vi "Config FX Set.vi"(5 "Max # Of Tries":i32, 6 "Send Cmd Timout(ms)":u32=300, 8 "Error":errorcluster, 9 "Wrist Config":T6={"WristHW Ver"=0, "CAN"={"ID"=0, "Bus"=""}, "Output"={"Type"=enum."Counter-Clockwise", "Neutral"=enum."EEPROMSetting", "Max"={"FWD"=0.0, "REV"=-1.0}, "Min"={"FWD"=0.0, "REV"=0.0}, "OL Ramp Rate (S)"=0.0, "Dead Band"=0.0}, "CL"={"Gains"={"P"=1.0, "I"=0.01, "D"=0.0, "F"=0.0}, "Error Allowed"={"High"=0.0, "Low"=0.0}, "I Zone"={"High"=10000.0, "Low"=-1000.0}, "Max Out"={"FWD"=1.0, "REV"=-1.0}, "Max I Accu"={"High"=10.0, "Low"=-10.0}, "CL Ramp Rate (S)"=0.0}, "MM"={"Cruise Velocity"=5000, "Acceleration"=5000}, "TravelLimits"={"Hard"={"FWD Switch Normal"=enum."Normally Open", "FWD On will Zero Encoder "=FALSE, "REV Switch Normal"=enum."Normally Open", "REV On will Zero Encoder "=FALSE}, "Soft"={"FWD"={"Enable"=FALSE, "Counts"=0}, "REV"={"Enable"=FALSE, "Counts"=0}}}, "Cancoder"={"ID"=0, "CW(t) CCW(f)"=TRUE, "Zero Offset"=0.0}, "CurrentLimit"={"Enable"=FALSE, "Current Limit"=0.0, "Threshold Current"=0.0, "Threshold Time"=0.0}} {"TravelLimits"."Soft"."REV"."Counts" format="%#.0f"; "TravelLimits"."Soft"."FWD"."Counts" format="%#.0f"; "Output"."Min"."REV" format="%.2f"; "Output"."Min"."FWD" format="%.2f"; "Output"."Max"."REV" format="%.2f"; "Output"."Max"."FWD" format="%.2f"; "CL"."Max I Accu"."Low" format="%#.8f"; "CL"."Max I Accu"."High" format="%#.8f"; "CL"."Gains"."F" format="%#.8f"; "CL"."Gains"."D" format="%#.8f"; "CL"."Gains"."I" format="%#.8f"; "CL"."Gains"."P" format="%#.8f"; "CL"."Error Allowed"."Low" format="%#.8f"; "CL"."Error Allowed"."High" format="%#.8f"; "CL"."I Zone"."Low" format="%#.8f"; "CL"."I Zone"."High" format="%#.8f"; "CL"."Max Out"."REV" format="%.2f"; "CL"."Max Out"."FWD" format="%.2f"}, 11 "PhoenixMotorControlDevRef":T1={"DeviceStatus"={"status"=FALSE, "code"=0, "source"=""}, "Type"=enum."PWM", "PWM"={"PWM Channel"=enum."Invalid", "DeadBand"={"Name"="", "maxPositivePwm"=0, "minPositivePwm"=0, "centerPwm"=0, "maxNegativePwm"=0, "minNegativePwm"=0, "angularRange"=0}}, "CAN"={"Device Number"=0, "SetOutput VI Ref"=variant, "GetOutput VI Ref"=variant, "Enable VI Ref"=variant, "Disable VI Ref"=variant, "Data"=variant}, "Invert"=FALSE, "DIO PWM"={"PWM \"Enable\" Channel"=enum."Invalid", "DIOChannel"=enum."Invalid", "PWM Rate"=0.0}}) -> (0 "Error Out":errorcluster, 3 "PhoenixMotorControlDevRef Out Out":T1)   [LabVIEW 2023, in "Wrist_ACT.lvlib"]
uses:
  Wrist_ACT.lvlib
  <vilib>/Utility/Data Type/NI_Data Type.lvlib
  Shared Code/TypeDefs/Cluser_CAN Data.ctl
  <vilib>/Rock Robotics/WPI/ThirdParty/Phoenix-LabVIEW/Motor Controller/Controls/CTRE_Phoenix_MotorControl_TalonFXInvertType.ctl
  <vilib>/Rock Robotics/WPI/ThirdParty/Phoenix-LabVIEW/Motor Controller/Controls/CTRE_Phoenix_MotorControl_NeutralMode.ctl
  Shared Code/TypeDefs/Cluster_FWD  REV Values.ctl
  Shared Code/TypeDefs/Cluster_Config Motor Output.ctl
  Shared Code/TypeDefs/Cluster_PID Gains.ctl
  Shared Code/TypeDefs/Cluster_High-Low.ctl
  Shared Code/TypeDefs/Cluster_PID Config.ctl
  Shared Code/TypeDefs/Cluster_Motion Magic Parameters.ctl
  <vilib>/Rock Robotics/WPI/ThirdParty/Phoenix-LabVIEW/Motor Controller/Controls/CTRE_Phoenix_MotorControl_LimitSwitchNormal.ctl
  Shared Code/TypeDefs/Cluser_Hard Limits.ctl
  Shared Code/TypeDefs/Cluser_Enable-Value I32.ctl
  Shared Code/TypeDefs/Cluser_Config_Soft Limits.ctl
  Shared Code/TypeDefs/Cluser_Limit Travel Config.ctl
  <vilib>/Rock Robotics/WPI/ThirdParty/Phoenix-LabVIEW/Motor Controller/Controls/CTRE_Phoenix_MotorControl_RemoteSourceType.ctl
  <vilib>/Rock Robotics/WPI/ThirdParty/Phoenix-LabVIEW/Motor Controller/Controls/CTRE_Phoenix_MotorControl_FeedbackDevice_TalonFX.ctl
  Shared Code/TypeDefs/Cluster_Config FX Motor Output.ctl
  Shared Code/TypeDefs/Cluster_FX SLOT PID Config.ctl
  <vilib>/Rock Robotics/SystemInterfaces/DIO/FPGA_DIOPWMChannel.ctl
  <vilib>/Rock Robotics/WPI/PWM/WPI_PWMDeadband.ctl
  <vilib>/Rock Robotics/WPI/MotorControl/WPI_MotorControlType.ctl
  <vilib>/Rock Robotics/SystemInterfaces/DIO/FPGA_DIOChannel.ctl
  <vilib>/Rock Robotics/WPI/MotorControl/WPI_MotorControlDeviceRef.ctl
  Shared Code/TypeDefs/Cluster_Wrist_Config HW Values.ctl
  Shared Code/TypeDefs/Cluster_Config_Cancoder Data.ctl
  Shared Code/TypeDefs/Cluser_Config_Current Limits.ctl
panel:
  # "Tune Output\nto 1023 Max"
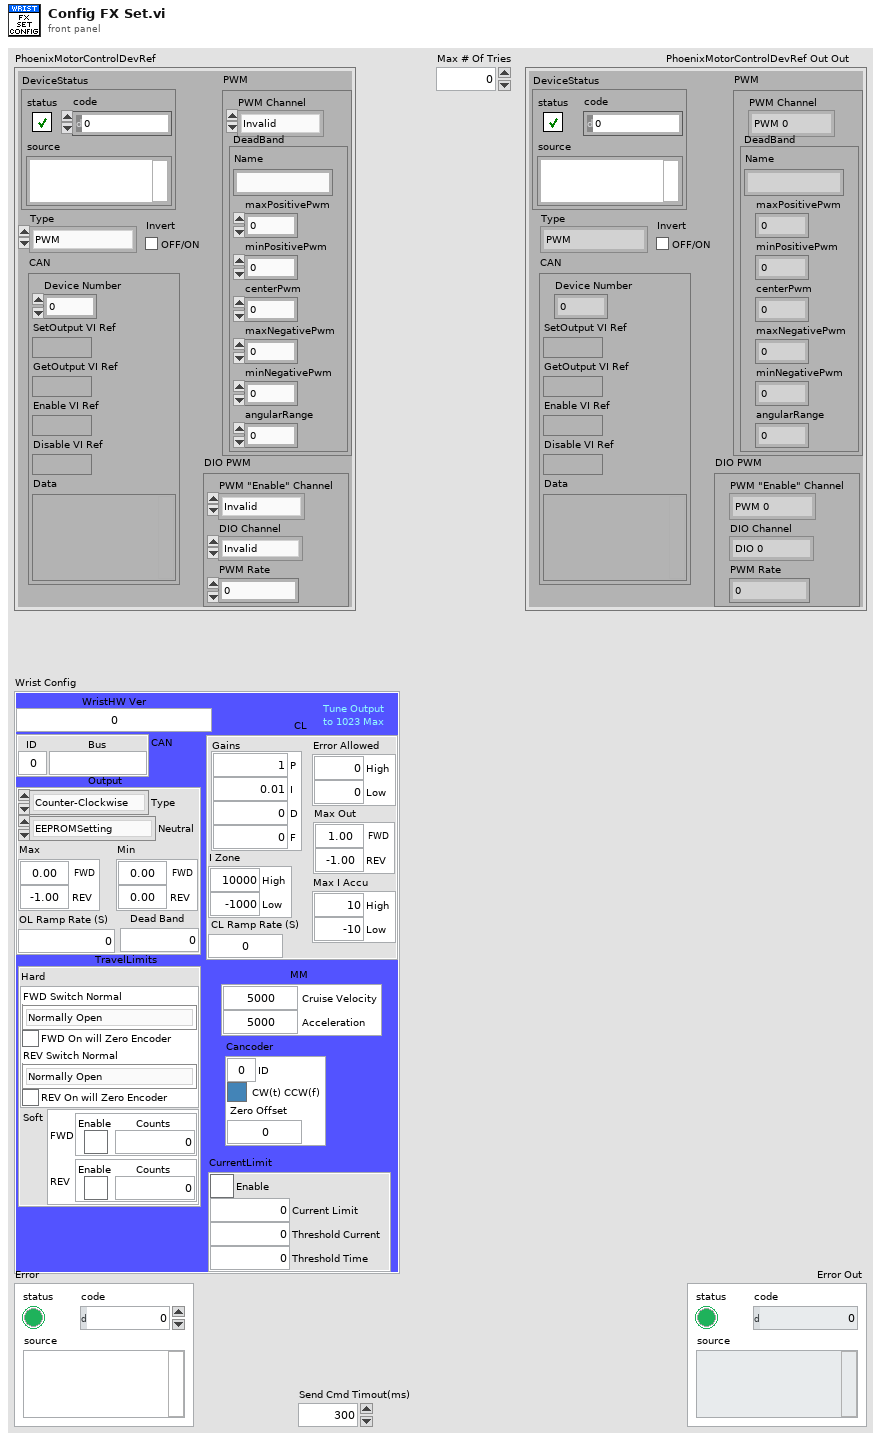
[diagram p1: front panel]
types:
  T1 = typedef "WPI_MotorControlDeviceRef.ctl" = cluster{"DeviceStatus":errorcluster, "Type":T2, "PWM":cluster{"PWM Channel":T3, "DeadBand":T4}, "CAN":cluster{"Device Number":u8, "SetOutput VI Ref":variant, "GetOutput VI Ref":variant, "Enable VI Ref":variant, "Disable VI Ref":variant, "Data":variant}, "Invert":bool, "DIO PWM":cluster{"PWM \"Enable\" Channel":T3, "DIOChannel":T5, "PWM Rate":dbl}}
  T2 = typedef "WPI_MotorControlType.ctl" = enum16{"PWM", "CAN", "DIO PWM"}
  T3 = typedef "FPGA_DIOPWMChannel.ctl" = enum8{"PWM 0", "PWM 1", "PWM 2", "PWM 3", "PWM 4", "PWM 5", "PWM 6", "PWM 7", "PWM 8", "PWM 9", "PWM MXP 0", "PWM MXP 1", "PWM MXP 2", "PWM MXP 3", "PWM MXP 4", "PWM MXP 5", "PWM MXP 6", "PWM MXP 7", "PWM MXP 8", "PWM MXP 9", "Invalid"}
  T4 = typedef "WPI_PWMDeadband.ctl" = cluster{"Name":string, "maxPositivePwm":i32, "minPositivePwm":i32, "centerPwm":i32, "maxNegativePwm":i32, "minNegativePwm":i32, "angularRange":u16}
  T5 = typedef "FPGA_DIOChannel.ctl" = enum8{"DIO 0", "DIO 1", "DIO 2", "DIO 3", "DIO 4", "DIO 5", "DIO 6", "DIO 7", "DIO 8", "DIO 9", "DIO MXP 0", "DIO MXP 1", "DIO MXP 2", "DIO MXP 3", "DIO MXP 4", "DIO MXP 5", "DIO MXP 6", "DIO MXP 7", "DIO MXP 8", "DIO MXP 9", "DIO MXP 10", "DIO MXP 11", "DIO MXP 12", "DIO MXP 13", "DIO MXP 14", "DIO MXP 15", "SPI Port CS1", "SPI Port CS2", "SPI Port CS3", "SPI Port MISO", "SPI Port MOSI", "Invalid"}
  T6 = typedef "Cluster_Wrist_Config HW Values.ctl" = cluster{"WristHW Ver":u64, "CAN":T7, "Output":T8, "CL":T12, "MM":T15, "TravelLimits":T16, "Cancoder":T21, "CurrentLimit":T22}
  T7 = typedef "Cluser_CAN Data.ctl" = cluster{"ID":u8, "Bus":string}
  T8 = typedef "Cluster_Config Motor Output.ctl" = cluster{"Type":T9, "Neutral":T10, "Max":T11, "Min":T11, "OL Ramp Rate (S)":dbl, "Dead Band":dbl}
  T9 = typedef "CTRE_Phoenix_MotorControl_TalonFXInvertType.ctl" = enum16{"Counter-Clockwise", "Clockwise"}
  T10 = typedef "CTRE_Phoenix_MotorControl_NeutralMode.ctl" = enum8{"EEPROMSetting", "Override to Coast", "Override to Brake"}
  T11 = typedef "Cluster_FWD  REV Values.ctl" = cluster{"FWD":dbl, "REV":dbl}
  T12 = typedef "Cluster_PID Config.ctl" = cluster{"Gains":T13, "Error Allowed":T14, "I Zone":T14, "Max Out":T11, "Max I Accu":T14, "CL Ramp Rate (S)":dbl}
  T13 = typedef "Cluster_PID Gains.ctl" = cluster{"P":dbl, "I":dbl, "D":dbl, "F":dbl}
  T14 = typedef "Cluster_High-Low.ctl" = cluster{"High":dbl, "Low":dbl}
  T15 = typedef "Cluster_Motion Magic Parameters.ctl" = cluster{"Cruise Velocity":i32, "Acceleration":i32}
  T16 = typedef "Cluser_Limit Travel Config.ctl" = cluster{"Hard":T17, "Soft":T19}
  T17 = typedef "Cluser_Hard Limits.ctl" = cluster{"FWD Switch Normal":T18, "FWD On will Zero Encoder ":bool, "REV Switch Normal":T18, "REV On will Zero Encoder ":bool}
  T18 = typedef "CTRE_Phoenix_MotorControl_LimitSwitchNormal.ctl" = enum16{"Normally Open", "Normally Closed", "Disabled"}
  T19 = typedef "Cluser_Config_Soft Limits.ctl" = cluster{"FWD":T20, "REV":T20}
  T20 = typedef "Cluser_Enable-Value I32.ctl" = cluster{"Enable":bool, "Counts":i32}
  T21 = typedef "Cluster_Config_Cancoder Data.ctl" = cluster{"ID":u8, "CW(t) CCW(f)":bool, "Zero Offset":dbl}
  T22 = typedef "Cluser_Config_Current Limits.ctl" = cluster{"Enable":bool, "Current Limit":dbl, "Threshold Current":dbl, "Threshold Time":dbl}
  T23 = typedef "Cluster_FX SLOT PID Config.ctl" = cluster{"Gains":T13, "Error Allowed":dbl, "I Zone":dbl, "Peak Out 0-1":dbl, "Max I Accu":dbl}
  T24 = typedef "Cluster_Config FX Motor Output.ctl" = cluster{"Type":T9, "Neutral":T10, "Max":T11, "Min":T11, "OL Ramp Rate (S)":dbl, "Dead Band":dbl, "CL Ramp Rate (S)":dbl}
  T25 = typedef "CTRE_Phoenix_MotorControl_RemoteSourceType.ctl" = enum16{"Off", "Talon SRX Selected Sensor", "Pigeon IMU Yaw", "Pigeon IMU Pitch", "Pigeon IMU Roll", "CANifier Quadrature", "CANifier PWM Input 0", "CANifier PWM Input 1", "CANifier PWM Input 2", "CANifier PWM Input 3", "Gadgeteer Pigeon Yaw", "Gadgeteer Pigeon Pitch", "Gadgeteer Pigeon Roll", "CANCoder"}
  T26 = typedef "CTRE_Phoenix_MotorControl_FeedbackDevice_TalonFX.ctl" = i8
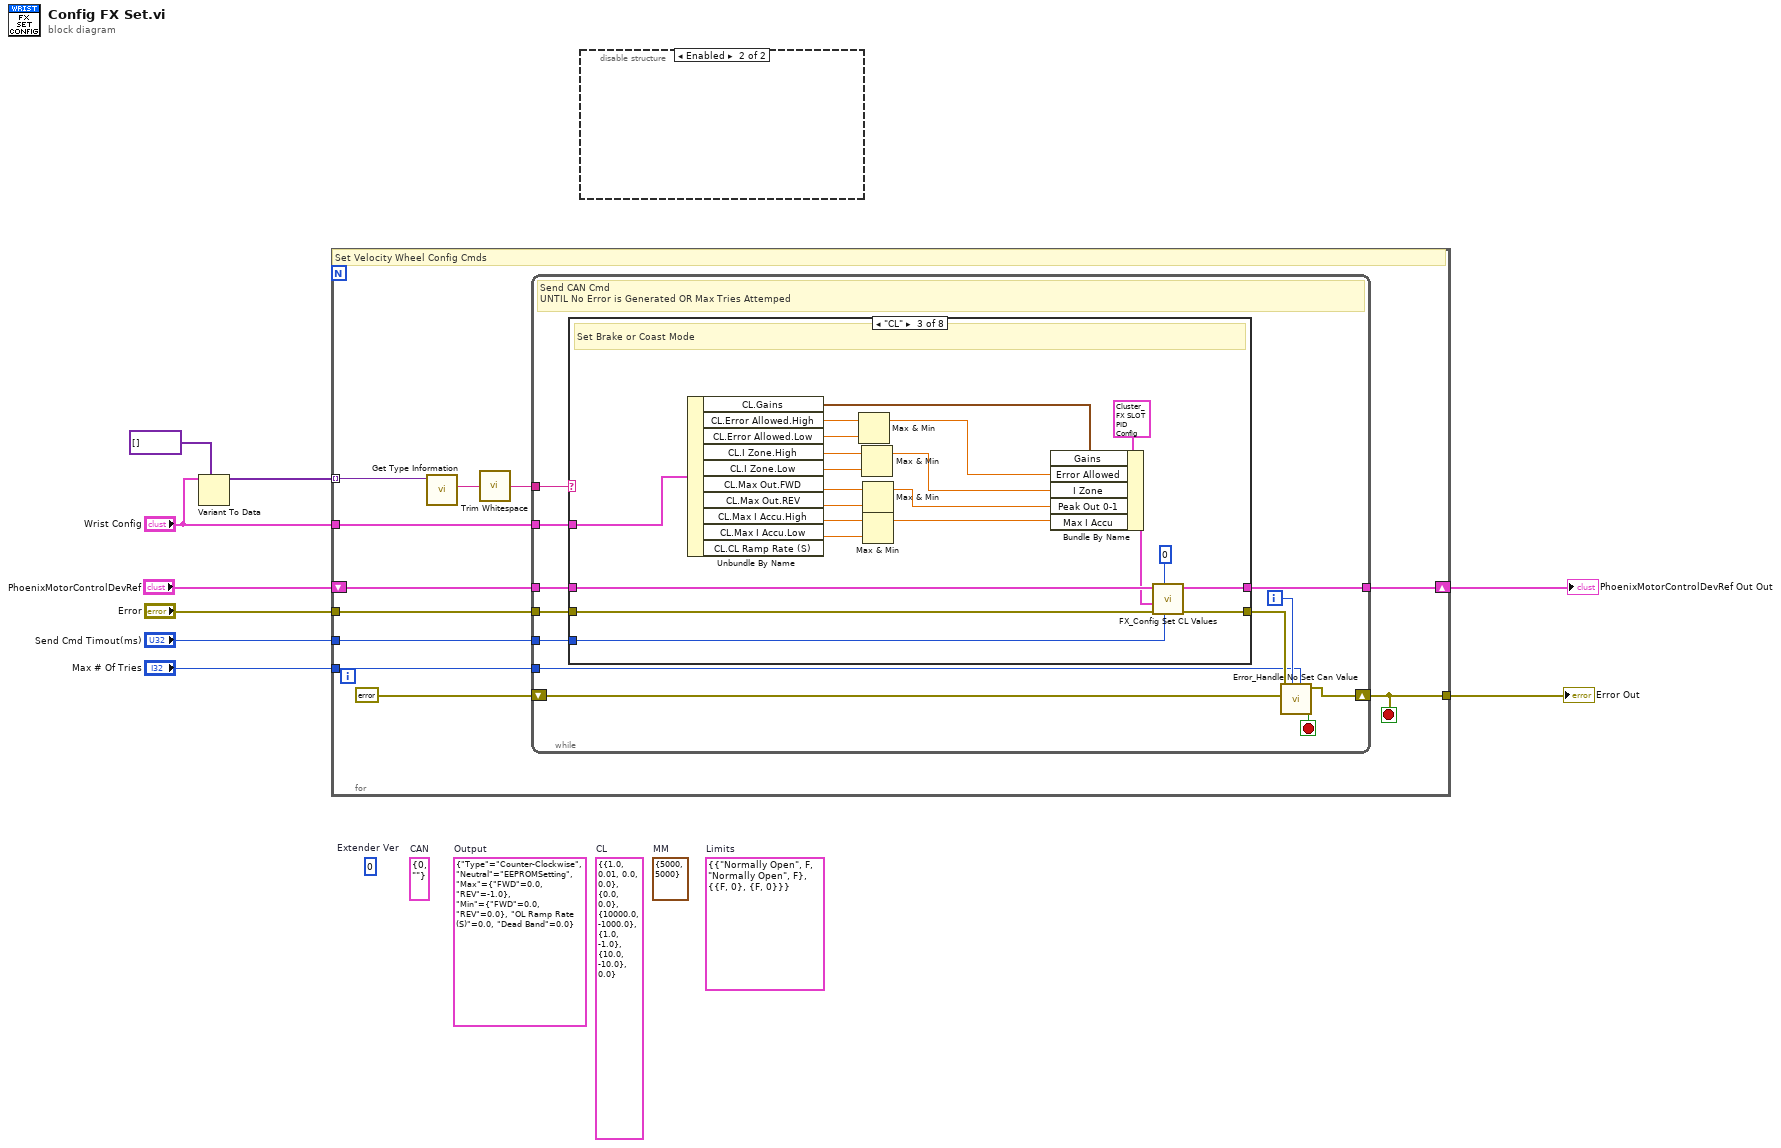
[diagram p0: block diagram]
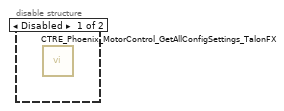
[diagram p2: hidden frame]
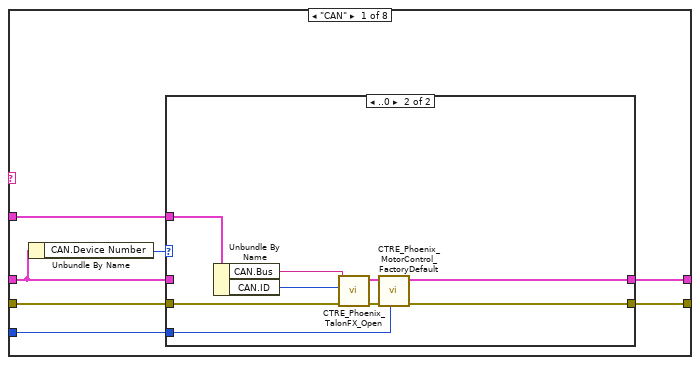
[diagram p3: hidden frame]
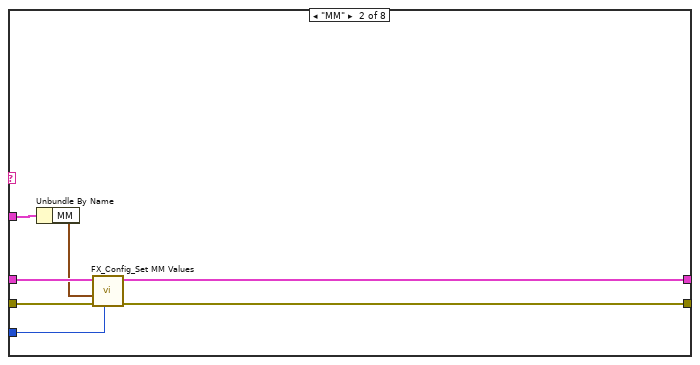
[diagram p5: hidden frame]
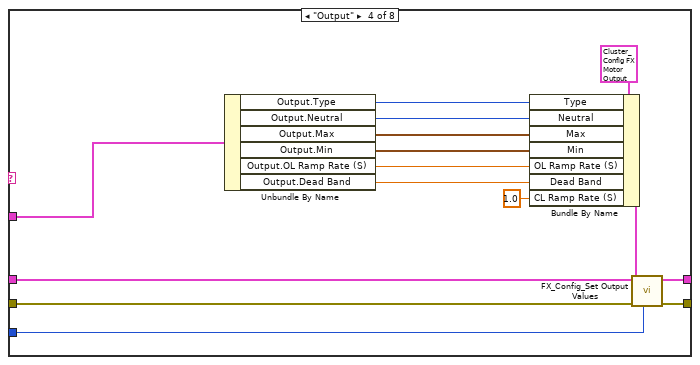
[diagram p6: hidden frame]
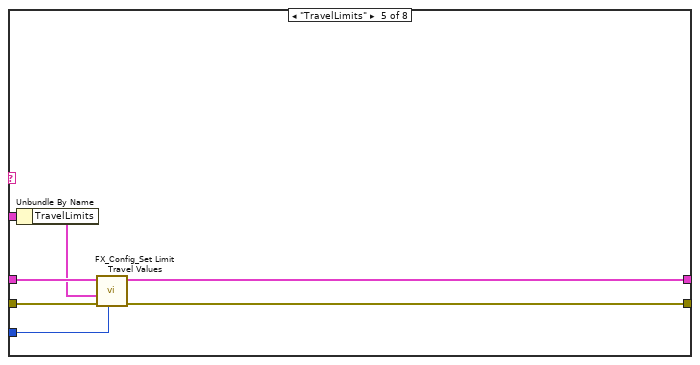
[diagram p7: hidden frame]
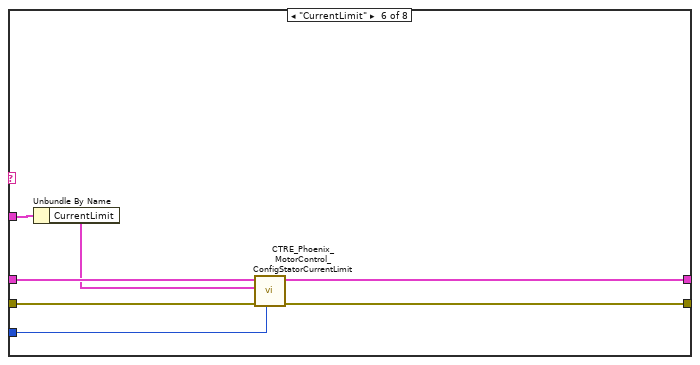
[diagram p8: hidden frame]
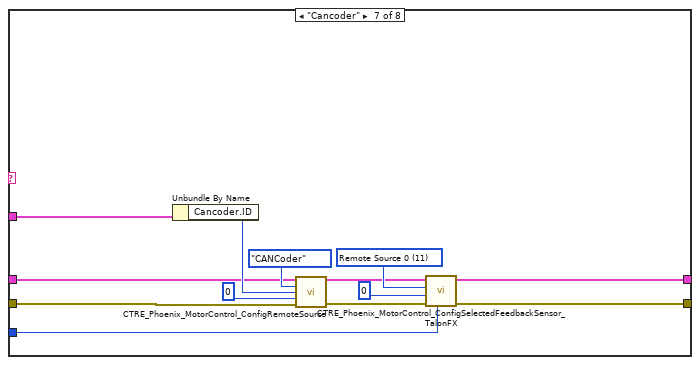
[diagram p9: hidden frame]
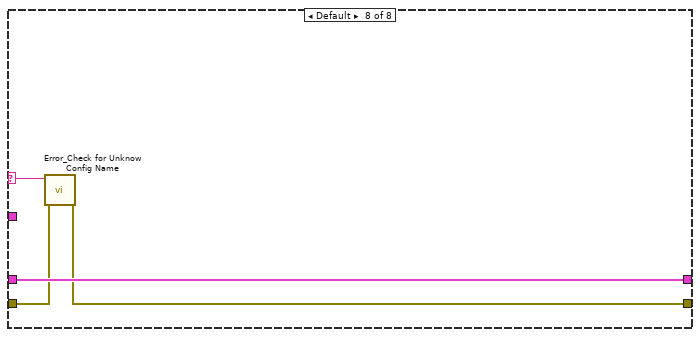
[diagram p10: hidden frame]
diagram:
  (unwired) T16 {"Hard"={"FWD Switch Normal"=enum."Normally Open", "FWD On will Zero Encoder "=FALSE, "REV Switch Normal"=enum."Normally Open", "REV On will Zero Encoder "=FALSE}, "Soft"={"FWD"={"Enable"=FALSE, "Counts"=0}, "REV"={"Enable"=FALSE, "Counts"=0}}}  # Limits
  (unwired) T15 {"Cruise Velocity"=5000, "Acceleration"=5000}  # MM
  (unwired) T12 {"Gains"={"P"=1.0, "I"=0.01, "D"=0.0, "F"=0.0}, "Error Allowed"={"High"=0.0, "Low"=0.0}, "I Zone"={"High"=10000.0, "Low"=-1000.0}, "Max Out"={"FWD"=1.0, "REV"=-1.0}, "Max I Accu"={"High"=10.0, "Low"=-10.0}, "CL Ramp Rate (S)"=0.0}  # CL
  (unwired) T8 {"Type"=enum."Counter-Clockwise", "Neutral"=enum."EEPROMSetting", "Max"={"FWD"=0.0, "REV"=-1.0}, "Min"={"FWD"=0.0, "REV"=0.0}, "OL Ramp Rate (S)"=0.0, "Dead Band"=0.0}  # Output
  (unwired) T7 {"ID"=0, "Bus"=""}  # CAN
  (unwired) u64 0  # Extender Ver
  n1 = Variant To Data(type=variant[] [] ("appended array"), Variant="Wrist Config") -> (data=w1:variant[])  [unwired: 1 in, 1 out]
  n2 = for {
    tunnel: "Send Cmd Timout(ms)" -> [w19]
    shift-right: [w20] -> w6
    shift-left: "PhoenixMotorControlDevRef" -> [w17]
    tunnel: "Wrist Config" -> [w18]
    tunnel: "Max # Of Tries" -> [w15]
    tunnel: w1 -> [w14] mode=indexing
    tunnel: "Error" -> [w16]
    tunnel: [w13] -> w5
    stop <- w13 stop-if-true
    # "Set Velocity Wheel Config Cmds"
    n3 = call <vilib>:"Get Type Information.vi"("variant"=w14) -> ("name"=w11:string)  [unwired: 6 in, 4 out]
    n4 = call <vilib>:"Trim Whitespace.vi"("string"=w11) -> ("trimmed string"=w10:string)  [unwired: 1 in]
    n5 = while {
      tunnel: [w24] -> w20
      tunnel: w19 -> [w30]
      shift-right: [w31] -> w13
      shift-left: errorcluster {"status"=FALSE, "code"=0, "source"=""} ("Error Out") -> [w29]
      tunnel: w16 -> [w27]
      tunnel: w17 -> [w26]
      tunnel: w18 -> [w25]
      tunnel: w15 -> [w23]
      tunnel: w10 -> [w22]
      i -> [w28]
      stop <- w21 stop-if-true
      # "Send CAN Cmd\nUNTIL No Error is Generated OR Max Tries Attemped"
      n6 = case shown="\"CL\"" w22 {
        selector: w22 -> [_ _ _ _ _ _ _ w124]
        tunnel: [w39 w56 w77 w92 w99 w102 w114 w122] -> w32
        tunnel: w30 -> [w37 w55 w73 w90 w97 w104 w112 _]
        tunnel: w27 -> [w38 w57 w76 w91 w98 w103 w113 w123]
        tunnel: w26 -> [w35 w54 w79 w93 w100 w108 w111 w125]
        tunnel: w25 -> [w33 w53 w75 w89 w96 w106 w109 _]
        tunnel: [w34 w52 w78 w94 w101 w107 w110 w125] -> w24
        frame "CAN" {
          n7 = Unbundle By Name(w35) -> ("CAN.Device Number"=w36:u8)
          n8 = case shown="..0" w36 {
            tunnel: [w40 w47] -> w39
            tunnel: w38 -> [w40 w46]
            tunnel: w37 -> [_ w45]
            tunnel: w35 -> [w41 _]
            tunnel: [w41 w43] -> w34
            tunnel: w33 -> [_ w42]
            frame 1.. {
            }
            frame ..0 {
              n9 = Unbundle By Name(w42) -> ("CAN.Bus"=w44:string, "CAN.ID"=w48:u8)
              n10 = call <vilib>:"CTRE_Phoenix_TalonFX_Open.vi"("error in"=w46, "Device Number"=w48, "CAN Bus"=w44) -> ("error out"=w49:errorcluster, "PhoenixMotorControlDevRef"=w50:T1)  [unwired: 7 in]
              n11 = call <vilib>:"CTRE_Phoenix_MotorControl_FactoryDefault.vi"("timeoutMs"=w45, "error in"=w49, "PhoenixMotorControlDevRef"=w50) -> ("error out"=w47:errorcluster, "PhoenixMotorControlDevRef"=w43:T1)  [unwired: 7 in]
            }
          }
        }
        frame "MM" {
          n12 = Unbundle By Name(w53) -> ("MM"=w51:T15)
          n13 = call "FX_Config_Set MM Values.vi"("Send Cmd Timout(ms)"=w55, "Error"=w57, "MM"=w51, "PhoenixMotorControlDevRef"=w54) -> ("Error Out"=w56:errorcluster, "PhoenixMotorControlDevRef Out"=w52:T1)  [unwired: 6 in]
        }
        frame "CL" {
          # "Set Brake or Coast Mode"
          n14 = Unbundle By Name(w75) -> ("CL.Gains"=w70:T13, "CL.Error Allowed.High"=w69:dbl, "CL.Error Allowed.Low"=w68:dbl, "CL.I Zone.High"=w67:dbl, "CL.I Zone.Low"=w66:dbl, "CL.Max Out.FWD"=w65:dbl, "CL.Max Out.REV"=w64:dbl, "CL.Max I Accu.High"=w63:dbl, "CL.Max I Accu.Low"=w62:dbl)  [unwired: 1 out]
          n15 = Max & Min(x=w69, y=w68) -> (max(x,y)=w61:dbl)  [unwired: 1 out]
          n16 = Max & Min(x=w67, y=w66) -> (max(x,y)=w60:dbl)  [unwired: 1 out]
          n17 = Max & Min(x=w65, y=w64) -> (max(x,y)=w59:dbl)  [unwired: 1 out]
          n18 = Max & Min(x=w63, y=w62) -> (max(x,y)=w58:dbl)  [unwired: 1 out]
          n19 = Bundle By Name(cluster=T23 {"Gains"={"P"=0.0, "I"=0.0, "D"=0.0, "F"=0.0}, "Error Allowed"=0.0, "I Zone"=0.0, "Peak Out 0-1"=0.0, "Max I Accu"=0.0} ("CL"), "Gains"=w70, "Error Allowed"=w61, "I Zone"=w60, "Peak Out 0-1"=w59, "Max I Accu"=w58) -> (w72:T23)
          n20 = call "FX_Config Set CL Values.vi"("Send Cmd Timout(ms)"=w73, "SlotIdx"=0, "Error"=w76, "CL"=w72, "PhoenixMotorControlDevRef"=w79) -> ("Error Out"=w77:errorcluster, "PhoenixMotorControlDevRef Out"=w78:T1)  [unwired: 4 in, 1 out]
        }
        frame "Output" {
          n21 = Unbundle By Name(w89) -> ("Output.Type"=w86:T9, "Output.Neutral"=w85:T10, "Output.Max"=w84:T11, "Output.Min"=w83:T11, "Output.OL Ramp Rate (S)"=w82:dbl, "Output.Dead Band"=w81:dbl)
          n22 = Bundle By Name(cluster=T24 {"Type"=enum."Counter-Clockwise", "Neutral"=enum."EEPROMSetting", "Max"={"FWD"=0.0, "REV"=0.0}, "Min"={"FWD"=0.0, "REV"=0.0}, "OL Ramp Rate (S)"=0.0, "Dead Band"=0.0, "CL Ramp Rate (S)"=0.0} ("Output"), "Type"=w86, "Neutral"=w85, "Max"=w84, "Min"=w83, "OL Ramp Rate (S)"=w82, "Dead Band"=w81, "CL Ramp Rate (S)"=1.0) -> (w87:T24)
          n23 = call "FX_Config_Set Output Values.vi"("Send Cmd Timout(ms)"=w90, "Error"=w91, "Output"=w87, "PhoenixMotorControlDevRef"=w93) -> ("Error Out"=w92:errorcluster, "PhoenixMotorControlDevRef Out"=w94:T1)  [unwired: 6 in]
        }
        frame "TravelLimits" {
          n24 = Unbundle By Name(w96) -> ("TravelLimits"=w95:T16)
          n25 = call "FX_Config_Set Limit Travel Values.vi"("Send Cmd Timout(ms)"=w97, "Error"=w98, "Limits"=w95, "PhoenixMotorControlDevRef"=w100) -> ("Error Out"=w99:errorcluster, "PhoenixMotorControlDevRef Out"=w101:T1)  [unwired: 6 in]
        }
        frame "CurrentLimit" {
          n26 = Unbundle By Name(w106) -> ("CurrentLimit"=w105:T22)
          n27 = call <vilib>:"CTRE_Phoenix_MotorControl_ConfigStatorCurrentLimit.vi"("timeoutMs"=w104, "error in (no error)"=w103, "Stator Current Limit Configuration"=w105, "PhoenixMotorControlDevRef"=w108) -> ("error out"=w102:errorcluster, "PhoenixMotorControlDevRef"=w107:T1)  [unwired: 6 in]
        }
        frame "Cancoder" {
          w118 = T26 11 items=["Integrated Sensor"=1, "Sensor Sum (S0 + S1)"=9, "Sensor Difference (D0 - D1)"=10, "Remote Source 0"=11, "Remote Source 1"=12, "None"=14, "Software Emulated"=15] ("Talon FX Feedback Device")
          n28 = Unbundle By Name(w109) -> ("Cancoder.ID"=w119:u8)
          n29 = call <vilib>:"CTRE_Phoenix_MotorControl_ConfigRemoteSource.vi"("PhoenixMotorControlDevRef"=w111, "Remote Device Type"=CTRE_Phoenix_MotorControl_RemoteSourceType."CANCoder", "Remote Device ID"=w119, "Source Index (0/1)"=u32 0, "error in (no error)"=w113) -> ("PhoenixMotorControlDevRef"=w115:T1, "error out"=w116:errorcluster)  [unwired: 9 in]
          n30 = call <vilib>:"CTRE_Phoenix_MotorControl_ConfigSelectedFeedbackSensor_TalonFX.vi"("timeoutMs"=w112, "error in (no error)"=w116, "pidLoopIdx"=0, "Talon FX Feedback Device"=w118, "PhoenixMotorControlDevRef"=w115) -> ("error out"=w114:errorcluster, "PhoenixMotorControlDevRef"=w110:T1)  [unwired: 5 in]
        }
        frame Default {
          n31 = call "Error_Check for Unknow Config Name.vi"("error in (no error)"=w123, "Config Name"=w124) -> ("error out"=w122:errorcluster)  [unwired: 9 in]
        }
      }
      n32 = call "Error_Handle No Set Can Value.vi"("Max # Of Tries"=w23, "Loop Itteration"=w28, "Previous Error"=w29, "Error"=w32) -> ("Stop Out"=w21:bool, "Error Out"=w31:errorcluster)  [unwired: 6 in]
    }
  }
  "Error Out" <- w5
  "PhoenixMotorControlDevRef Out Out" <- w6
  n33 = disable-structure shown="Enabled" {
    frame Disabled {
      n34 = call <vilib>:"CTRE_Phoenix_MotorControl_GetAllConfigSettings_TalonFX.vi"() -> ()  [unwired: 9 in, 3 out]
    }
    frame Enabled {
    }
  }
